vi "Add Rows.vi"   [LabVIEW 2016, in "DataGrid.lvlib" / "DataTable.lvclass"]
uses:
  <userlib>/LabVIEWdotNetDataGrid/source/DataTable/DataTable.lvclass
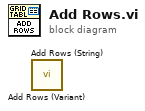
[diagram p0: block diagram]
diagram:
  n1 = call <userlib>:"Add Rows (Variant).vi"() -> ()  [unwired: 10 in, 2 out]
  n2 = call <userlib>:"Add Rows (String).vi"() -> ()  [unwired: 10 in, 2 out]
